vi "ThreeStateBooleanArray.vi"() -> ()   [LabVIEW 2018]
doc: "This VI demonstrates the creation and operation of a tri-state boolean array. The values are initialized to black and can then be changed to two other colors by clicking on the boolean.\n\nCopyright © 2011 Epimedia, Inc. All Rights Reserved.\n\nThe Epimedia Application Library is Copyright © 2009-2011 Epimedia, Inc. \nAll Rights Reserved. Used under license."
panel:
  out "32bit integer":i32
  out "ArrayIndex":i32
  out "ElementHeight":i32
  out "ElementTop":i32
  out "LED":u32[](array[colorbox]) caption="D1\nD2\nD3\nD4\nD5"
  out "ChkInStat":bool[](array[boolean])
  in  "stop":bool
  # "Copyright © 2011 Epimedia, Inc. All Rights Reserved.\n\nThe Epimedia Application Library is Copyright © 2009-2011 Epimedia, Inc. \nAll Rights Reserved. Used under license."
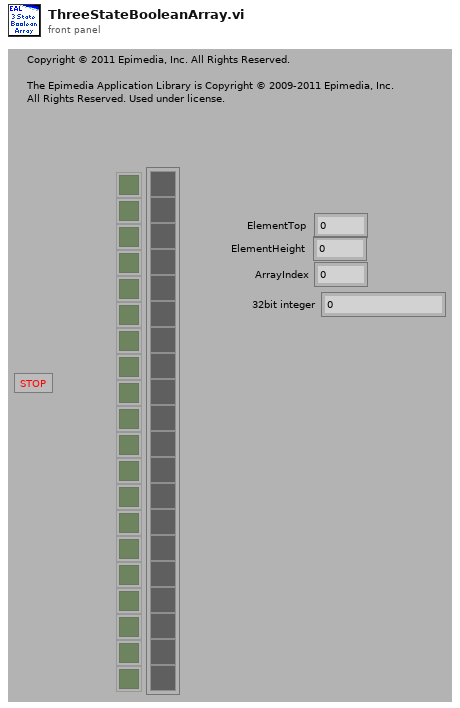
[diagram p1: front panel]
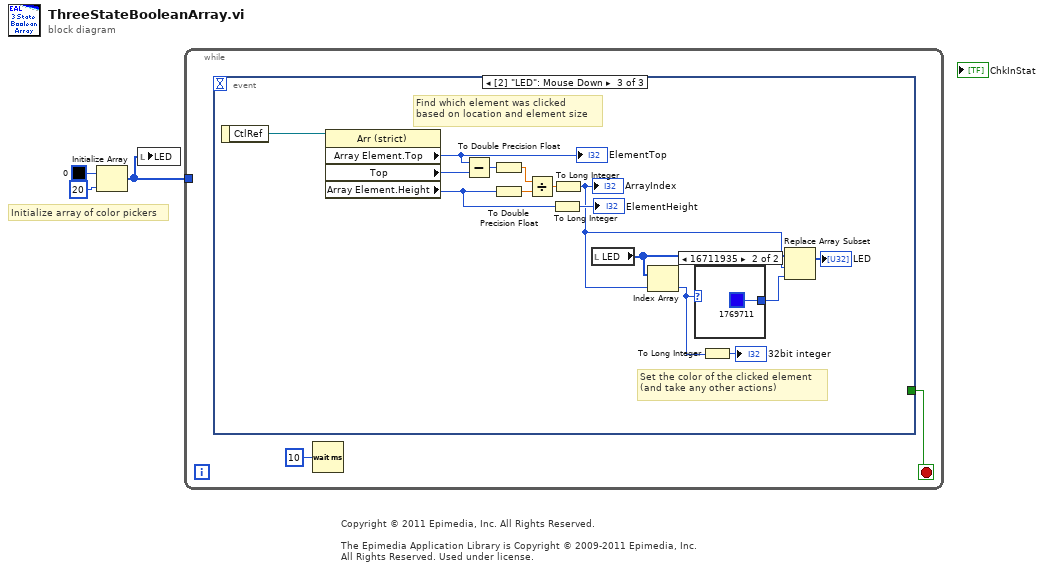
[diagram p0: block diagram]
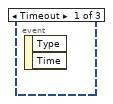
[diagram p2: hidden frame]
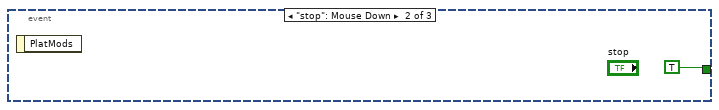
[diagram p3: hidden frame]
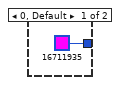
[diagram p4: hidden frame]
diagram:
  # "Copyright © 2011 Epimedia, Inc. All Rights Reserved.\n\nThe Epimedia Application Library is Copyright © 2009-2011 Epimedia, Inc. \nAll Rights Reserved. Used under license."
  # "Initialize array of color pickers"
  n1 = Initialize Array(u32 0, 20 ("dimension size")) -> (w1:u32[])
  n2 = local write "LED"(w1) -> ()
  n3 = while {
    tunnel: w1 -> [_]
    stop <- w4 stop-if-true
    n4 = event shown="[2] \"LED\": Mouse Down" {
      selector: _ -> [_ _ _]
      dyn-events: _ -> [_ _ _]
      timeout: _ -> [_ _ _]
      tunnel: [_ TRUE _] -> w4
      event Timeout {
        n5 = event-data() -> ()  [unwired: 1 in, 2 out]
      }
      event "stop": Mouse Down {
        n6 = event-data() -> ()  [unwired: 1 in, 1 out]
      }
      event "LED": Mouse Down {
        # "Set the color of the clicked element\n(and take any other actions)"
        # "Find which element was clicked\nbased on location and element size"
        n7 = event-data() -> ("CtlRef"=w21:refnum<vi>)  [unwired: 1 in]
        n8 = property class="Arr (strict)"(reference=w21) -> ("Array Element.Top"=w20:i32, "Top"=w18:i32, "Array Element.Height"=w17:u32)  [unwired: 1 in, 2 out]
        "ElementTop" <- w20
        n9 = Subtract(x=w20, y=w18) -> (x-y=w19:i32)
        n10 = To Double Precision Float(number=w19) -> (double precision float=w8:dbl)
        n11 = To Double Precision Float(number=w17) -> (double precision float=w7:dbl)
        n12 = Divide(x=w8, y=w7) -> (x/y=w12:dbl)
        n13 = To Long Integer(number=w17) -> (32bit integer=→"ElementHeight":i32)
        n14 = To Long Integer(number=w12) -> (32bit integer=w9:i32)
        "ArrayIndex" <- w9
        n15 = local read "LED"() -> (w13:u32[])
        n16 = Index Array(array=w13, index=w9) -> (element=w11:u32)
        n17 = case shown="16711935" w11 {
          tunnel: [u32 16711935 u32 1769711] -> w15
          frame 0, Default {
          }
          frame 16711935 {
          }
        }
        n18 = To Long Integer(number=w11) -> (32bit integer=→"32bit integer":i32)
        n19 = Replace Array Subset(array=w13, new element=w15, index=w9) -> (→"LED":u32[])
      }
    }
    n20 = Wait (ms)(milliseconds to wait=u32 10) -> ()  [unwired: 1 out]
  }
